vi "SP Interpolate Marker Values.vi"(6 "Marker Value":dbl, 8 "Y Values":dbl[](array[numeric]), 9 "X Values":dbl[](array[numeric])) -> (1 "Interpolated Y Value":dbl)   [LabVIEW 2011]
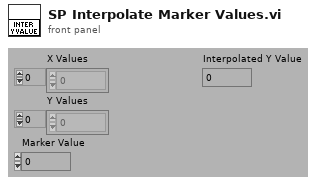
[diagram p1: front panel]
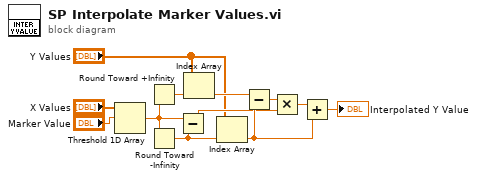
[diagram p0: block diagram]
diagram:
  n1 = Threshold 1D Array(2:"Marker Value", 3:"X Values") -> (0:w8:dbl)  [unwired: 1 out]
  n2 = Round Toward +Infinity(x=w8) -> (ceil(x): smallest int >= x=w7:dbl)
  n3 = Round Toward -Infinity(1:w8) -> (0:w6:dbl)
  n4 = Subtract(x=w8, y=w6) -> (x-y=w5:dbl)
  n5 = Index Array(array="Y Values", index=w7) -> (element=w12:dbl)
  n6 = Index Array(array="Y Values", index=w6) -> (element=w11:dbl)
  n7 = Subtract(x=w12, y=w11) -> (x-y=w10:dbl)
  n8 = Multiply(x=w10, y=w5) -> (x*y=w9:dbl)
  n9 = Add(x=w9, y=w11) -> (x+y=→"Interpolated Y Value":dbl)
